vi "Wrapper_getWavelengths_Mod.vi"(8 "error in (no error)":errorcluster caption="entrée d'erreur (pas d'erreur)", 10 "Wrapper":u32, 11 "Index":i32) -> (0 "error out":errorcluster caption="sortie d'erreur", 1 "Length":i32, 2 "WL Values":dbl[](array[numeric]))   [LabVIEW 2024]
uses:
  Program Files (x86)/Ocean Optics/OmniDriver/OOI_HOME/common32.dll
  Program Files (x86)/Ocean Optics/OmniDriver/OOI_HOME/OmniDriver32.dll
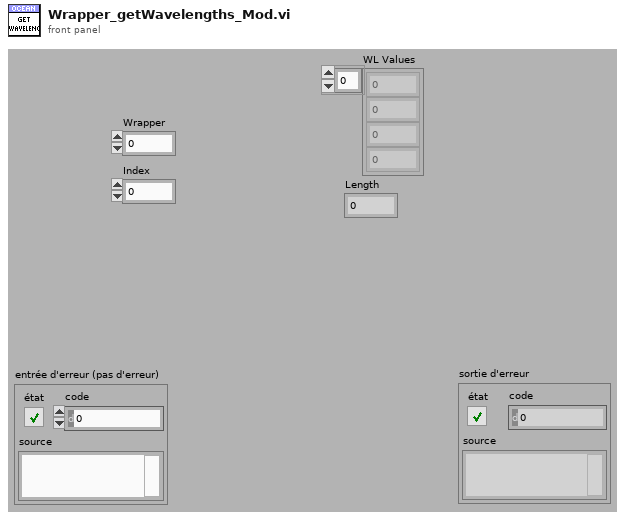
[diagram p1: front panel]
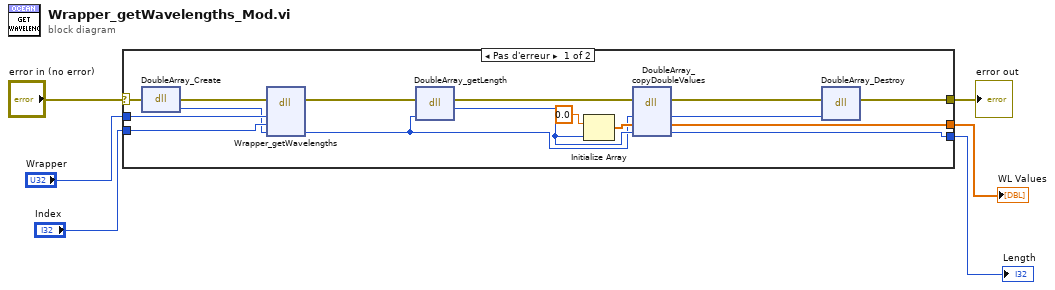
[diagram p0: block diagram]
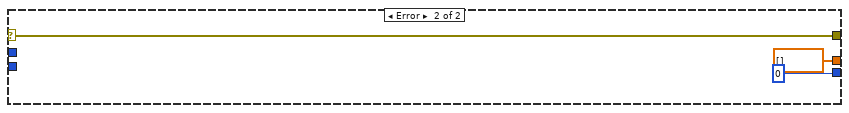
[diagram p2: hidden frame]
diagram:
  n1 = case shown="Pas d'erreur" "error in (no error)" {
    selector: "error in (no error)" -> [w12 w25]
    tunnel: "Wrapper" -> [w22 _]
    tunnel: "Index" -> [w21 _]
    tunnel: [w15 dbl[] [] ("Values")] -> w4
    tunnel: [w14 0 ("Length")] -> w3
    tunnel: [w7 w25] -> w1
    frame No Error {
      n2 = dll-call lib="C:/Program Files (x86)/Ocean Optics/OmniDriver/OOI_HOME/common32.dll" fn="DoubleArray_Create" label="DoubleArray.Create"(error in=w12) -> (error out=w11:errorcluster, "return type"=w20:u32)  [unwired: 2 in, 1 out]
      n3 = dll-call lib="C:/Program Files (x86)/Ocean Optics/OmniDriver/OOI_HOME/OmniDriver32.dll" fn="Wrapper_getWavelengths" label="Wrapper.getWavelengths"(error in=w11, "Wrapper"=w22, "Index"=w21, "WL DoubleArray"=w20) -> (error out=w10:errorcluster, "WL DoubleArray"=w16:u32)  [unwired: 4 in, 2 out]
      n4 = dll-call lib="C:/Program Files (x86)/Ocean Optics/OmniDriver/OOI_HOME/common32.dll" fn="DoubleArray_getLength" label="DoubleArray.getLength"(error in=w10, "DoubbleArray"=w16) -> (error out=w9:errorcluster, "return type"=w18:i32)  [unwired: 3 in, 1 out]
      n5 = Initialize Array(0.0 ("element"), w18) -> (w17:dbl[])
      n6 = dll-call lib="C:/Program Files (x86)/Ocean Optics/OmniDriver/OOI_HOME/common32.dll" fn="DoubleArray_copyDoubleValues" label="DoubleArray.coopyDoubleValues"(error in=w9, "DoubleArray"=w16, "Values"=w17, "Length"=w18) -> (error out=w8:errorcluster, "DoubleArray"=w13:u32, "Values"=w15:dbl[], "Length"=w14:i32)  [unwired: 2 in, 2 out]
      n7 = dll-call lib="C:/Program Files (x86)/Ocean Optics/OmniDriver/OOI_HOME/common32.dll" fn="DoubleArray_Destroy" label="DoubleArray.Destroy"(error in=w8, "DoubleArray"=w13) -> (error out=w7:errorcluster)  [unwired: 3 in, 2 out]
    }
    frame Error {
    }
  }
  "WL Values" <- w4
  "Length" <- w3
  "error out" <- w1
